vi "Pkg New.vi"(8 "error in (no error)":errorcluster, 10 "Package Name":string, 11 "Root Directory":path) -> (0 "error out":errorcluster, 3 "Created":path[](array[path]))   [LabVIEW 2018, in "Pkg.lvlib"]
uses:
  Pkg.lvlib
  <vilib>/ErrorRing/Error Ring.xnode
  <vilib>/Utility/error.llb/Error Cluster From Error Code.vi
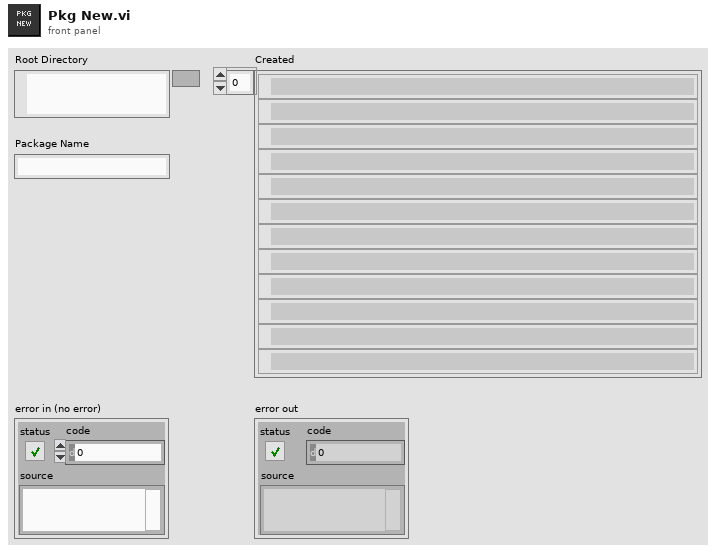
[diagram p1: front panel]
types:
  T1 = cluster{"RootDir":path, "PkgName":string, "PkgDir":path, "PkgBuildsDir":path, "PkgConfigsDir":path, "PkgDocsDir":path, "PkgLibDir":path, "PkgTestsDir":path, "PkgPackageIni":path, "PkgLibLvproj":path, "PkgLibSettingsIni":path, "PkgLibLvlib":path, "PkgLibVI":path}
  T2 = enum32{"invalid app kind", "Development System", "Run Time System", "Student Edition", "Embedded LabVIEW", "Evaluation", "Custom"}
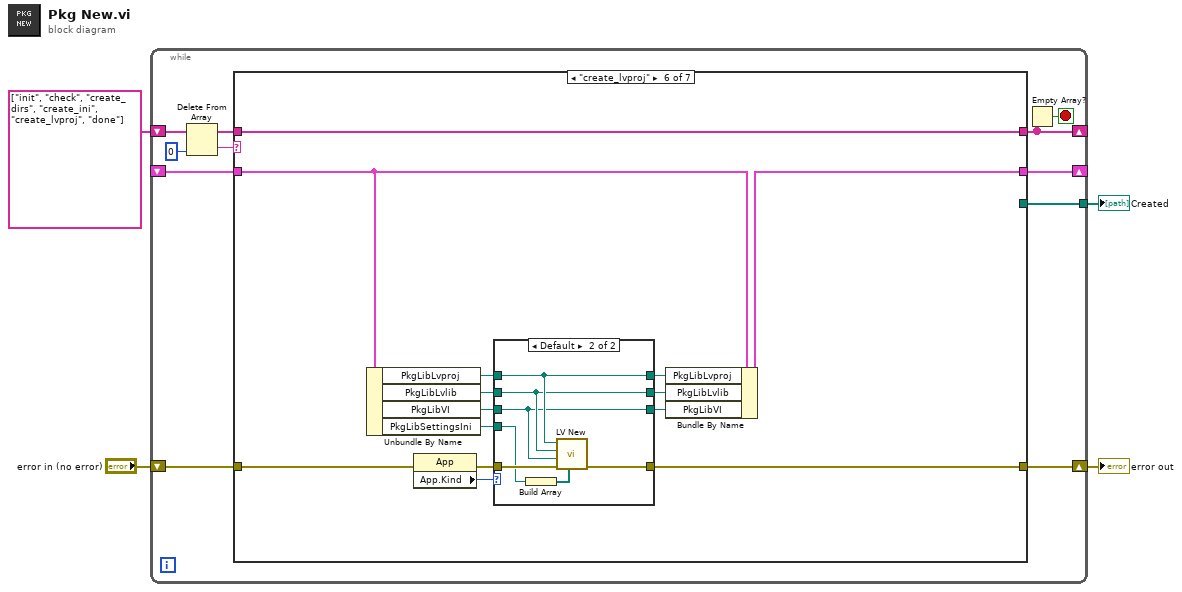
[diagram p0: block diagram]
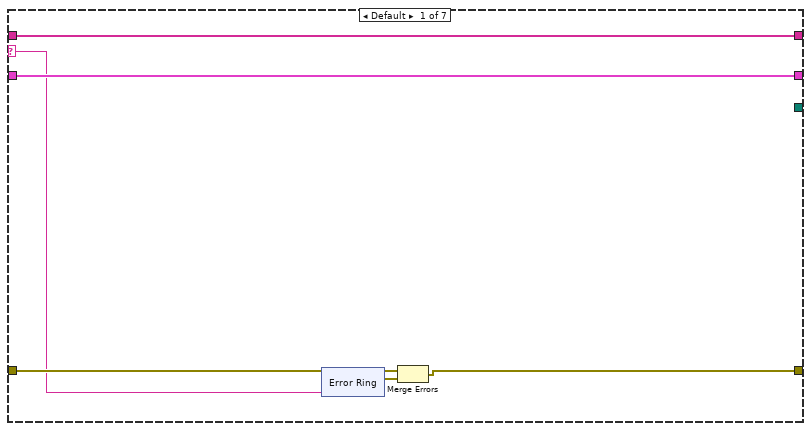
[diagram p2: hidden frame]
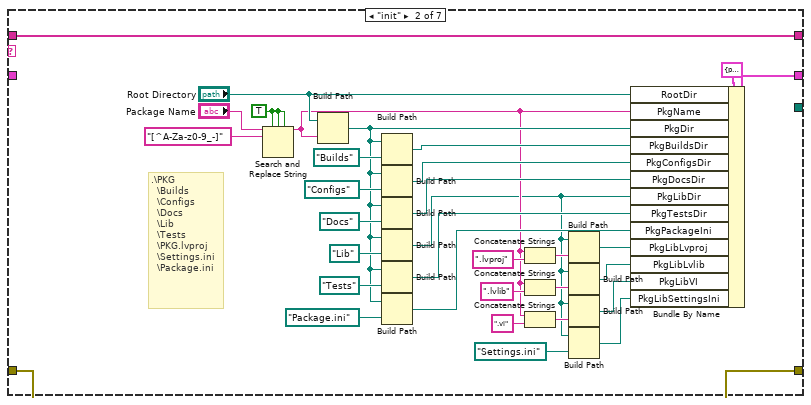
[diagram p3: hidden frame]
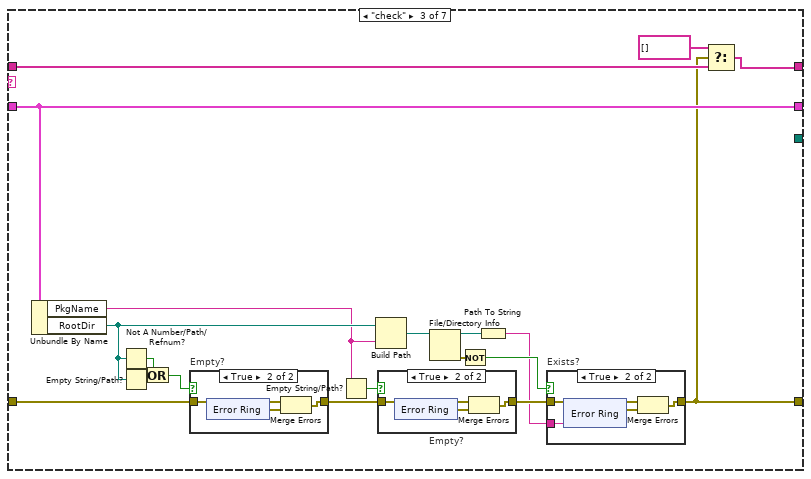
[diagram p4: hidden frame]
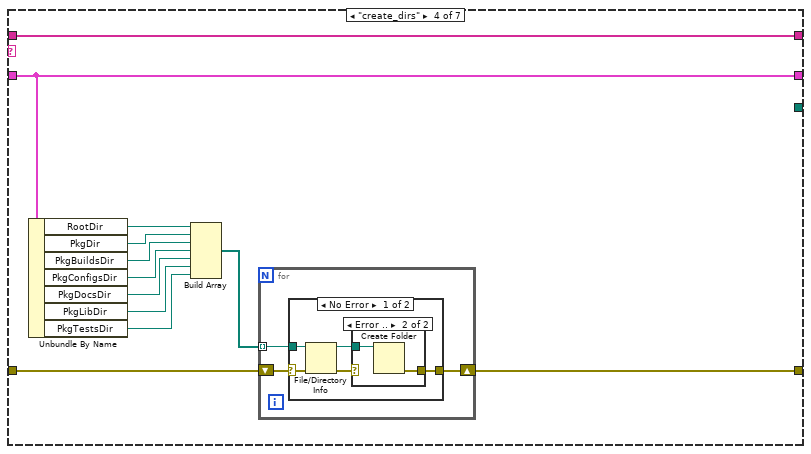
[diagram p8: hidden frame]
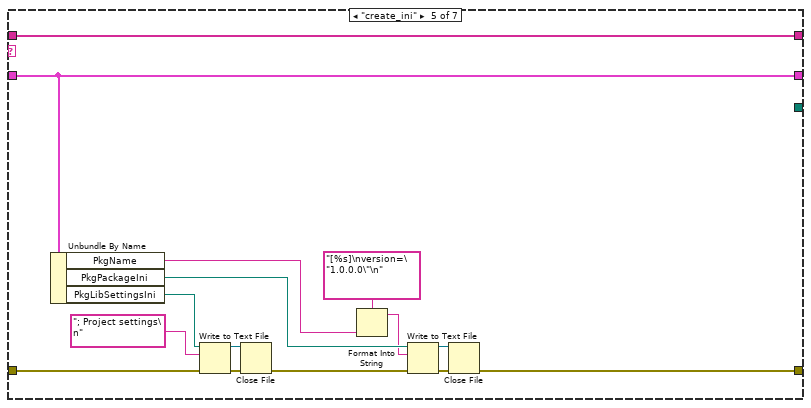
[diagram p11: hidden frame]
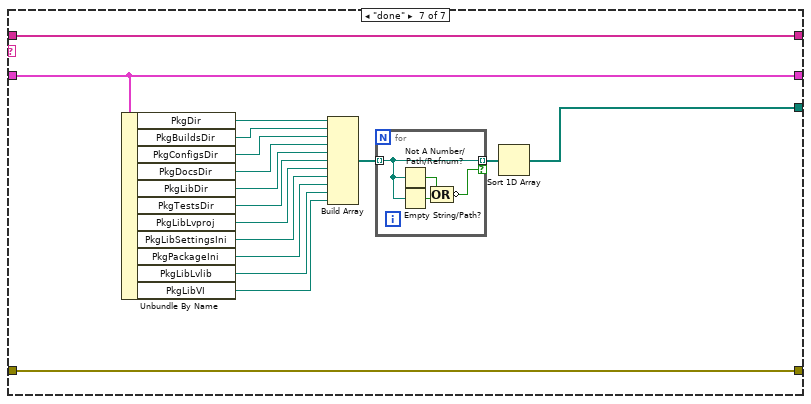
[diagram p13: hidden frame]
diagram:
  n1 = while {
    shift-right: [w7] -> _
    shift-left: string[] ["init", "check", "create_dirs", "create_ini", "create_lvproj", "done"] -> [w15]
    shift-right: [w9] -> _
    shift-left: _ -> [w8]
    shift-right: [w11] -> w3
    shift-left: "error in (no error)" -> [w10]
    tunnel: [w5] -> w1
    stop <- w6 stop-if-true
    n2 = Delete From Array(array=w15, index=0) -> (deleted portion=w12:string, array with subset deleted=w13:string[])  [unwired: 1 in]
    n3 = case shown="\"create_lvproj\"" w12 {
      selector: w12 -> [w16 _ _ _ _ _ _]
      tunnel: [w21 w61 w75 w122 w149 w163 w188] -> w7
      tunnel: w13 -> [w21 w61 w74 w122 w149 w163 w188]
      tunnel: [w18 w39 w64 w120 w139 w160 w187] -> w11
      tunnel: w10 -> [w19 w39 w80 w118 w148 w161 w187]
      tunnel: [w20 w59 w79 w121 w147 w154 w186] -> w9
      tunnel: w8 -> [w20 _ w79 w121 w147 w162 w186]
      tunnel: [_ _ _ _ _ _ w172] -> w5
      frame Default {
        n4 = xnode "Error Ring"("parameter 0"=w16) -> ("error out"=w17:errorcluster)
        n5 = Merge Errors(w19, w17) -> (w18:errorcluster)
      }
      frame "init" {
        w58 = TRUE ("replace all? (F)")
        # ".\\PKG\n  \\Builds\n  \\Configs\n  \\Docs\n  \\Lib\n  \\Tests\n  \\PKG.lvproj\n  \\Settings.ini\n  \\Package.ini"
        n6 = Search and Replace String(replace all?=w58, case sensitive?=w58, multiline?=w58, input string="Package Name", search string="[^A-Za-z0-9_-]") -> (result string=w32:string)  [unwired: 3 in, 3 out]
        n7 = Build Path(base path="Root Directory", name or relative path=w32) -> (appended path=w36:path)
        n8 = Build Path(base path=w36, name or relative path=path "Builds") -> (appended path=w49:path)
        n9 = Build Path(base path=w36, name or relative path=path "Configs") -> (appended path=w48:path)
        n10 = Build Path(base path=w36, name or relative path=path "Docs") -> (appended path=w47:path)
        n11 = Build Path(base path=w36, name or relative path=path "Lib") -> (appended path=w30:path)
        n12 = Build Path(base path=w36, name or relative path=path "Tests") -> (appended path=w46:path)
        n13 = Build Path(base path=w36, name or relative path=path "Package.ini") -> (appended path=w35:path)
        n14 = Concatenate Strings(w32, ".lvproj" ("string")) -> (w41:string)
        n15 = Concatenate Strings(w32, ".lvlib" ("string")) -> (w45:string)
        n16 = Concatenate Strings(w32, ".vi" ("string")) -> (w42:string)
        n17 = Build Path(base path=w30, name or relative path=w41) -> (appended path=w31:path)
        n18 = Build Path(base path=w30, name or relative path=w45) -> (appended path=w34:path)
        n19 = Build Path(base path=w30, name or relative path=w42) -> (appended path=w33:path)
        n20 = Build Path(base path=w30, name or relative path=path "Settings.ini") -> (appended path=w29:path)
        n21 = Bundle By Name(cluster=T1 {"RootDir"=path "", "PkgName"="", "PkgDir"=path "", "PkgBuildsDir"=path "", "PkgConfigsDir"=path "", "PkgDocsDir"=path "", "PkgLibDir"=path "", "PkgTestsDir"=path "", "PkgPackageIni"=path "", "PkgLibLvproj"=path "", "PkgLibSettingsIni"=path "", "PkgLibLvlib"=path "", "PkgLibVI"=path ""} ("StateData"), "RootDir"="Root Directory", "PkgName"=w32, "PkgDir"=w36, "PkgBuildsDir"=w49, "PkgConfigsDir"=w48, "PkgDocsDir"=w47, "PkgLibDir"=w30, "PkgTestsDir"=w46, "PkgPackageIni"=w35, "PkgLibLvproj"=w31, "PkgLibLvlib"=w34, "PkgLibVI"=w33, "PkgLibSettingsIni"=w29) -> (w59:T1)
      }
      frame "check" {
        n22 = Unbundle By Name(w79) -> ("PkgName"=w69:string, "RootDir"=w70:path)
        n23 = Not A Number/Path/Refnum?(number/path/refnum=w70) -> (NaN/Path/Refnum?=w77:bool)
        n24 = Empty String/Path?(string/path=w70) -> (empty?=w78:bool)
        n25 = Or(x=w77, y=w78) -> (x .or. y?=w73:bool)
        n26 = case "Empty?" shown="True" w73 {
          tunnel: w80 -> [w102 w105]
          tunnel: [w102 w103] -> w72
          frame False {
          }
          frame True {
            n27 = xnode "Error Ring"() -> ("error out"=w104:errorcluster)
            n28 = Merge Errors(w105, w104) -> (w103:errorcluster)
          }
        }
        n29 = Empty String/Path?(string/path=w69) -> (empty?=w71:bool)
        n30 = Build Path(base path=w70, name or relative path=w69) -> (appended path=w68:path)
        n31 = case "Empty?" shown="True" w71 {
          tunnel: w72 -> [w93 w96]
          tunnel: [w93 w94] -> w65
          frame False {
          }
          frame True {
            n32 = xnode "Error Ring"() -> ("error out"=w95:errorcluster)
            n33 = Merge Errors(w96, w95) -> (w94:errorcluster)
          }
        }
        n34 = File/Directory Info(path=w68) -> (path out=w63:path, error out=w67:errorcluster)  [unwired: 1 in, 5 out]
        n35 = Not(x=w67) -> (.not. x?=w66:bool)
        n36 = Path To String(path=w63) -> (string=w62:string)
        n37 = case "Exists?" shown="True" w66 {
          tunnel: w65 -> [w81 w85]
          tunnel: [w81 w83] -> w64
          tunnel: w62 -> [_ w82]
          frame False {
          }
          frame True {
            n38 = xnode "Error Ring"("parameter 0"=w82) -> ("error out"=w84:errorcluster)
            n39 = Merge Errors(w85, w84) -> (w83:errorcluster)
          }
        }
        n40 = Select(t=string[] [], s=w64, f=w74) -> (s? t:f=w75:string[])
      }
      frame "create_dirs" {
        n41 = Unbundle By Name(w121) -> ("RootDir"=w119:path, "PkgDir"=w116:path, "PkgBuildsDir"=w115:path, "PkgConfigsDir"=w114:path, "PkgDocsDir"=w113:path, "PkgLibDir"=w112:path, "PkgTestsDir"=w111:path)
        n42 = Build Array(w119, w116, w115, w114, w113, w112, w111) -> (w117:path[])
        n43 = for {
          tunnel: w117 -> [w124] mode=indexing
          shift-right: [w125] -> w120
          shift-left: w118 -> [w123]
          n44 = case shown="No Error" w123 {
            selector: w123 -> [w126 w134]
            tunnel: [w130 w134] -> w125
            tunnel: w124 -> [w129 _]
            frame No Error {
              n45 = File/Directory Info(path=w129, error in=w126) -> (path out=w128:path, error out=w127:errorcluster)  [unwired: 5 out]
              n46 = case shown="Error .." w127 {
                selector: w127 -> [w131 _]
                tunnel: [w131 w133] -> w130
                tunnel: w128 -> [_ w132]
                frame No Error {
                }
                frame Error {
                  n47 = Create Folder(path (use dialog)=w132) -> (error out=w133:errorcluster)  [unwired: 2 in, 2 out]
                }
              }
            }
            frame Error {
            }
          }
        }
      }
      frame "create_ini" {
        n48 = Unbundle By Name(w147) -> ("PkgName"=w136:string, "PkgPackageIni"=w138:path, "PkgLibSettingsIni"=w144:path)
        n49 = Write to Text File(file (use dialog)=w144, text="; Project settings\n", error in=w148) -> (refnum out=w145:refnum<file>, error out=w146:errorcluster)  [unwired: 1 in, 1 out]
        n50 = Close File(refnum=w145, error in=w146) -> (error out=w140:errorcluster)  [unwired: 1 out]
        n51 = Format Into String(format string="[%s]\nversion=\"1.0.0.0\"\n" ("text"), w136) -> (resulting string=w135:string)  [unwired: 2 in, 1 out]
        n52 = Write to Text File(file (use dialog)=w138, text=w135, error in=w140) -> (refnum out=w142:refnum<file>, error out=w141:errorcluster)  [unwired: 1 in, 1 out]
        n53 = Close File(refnum=w142, error in=w141) -> (error out=w139:errorcluster)  [unwired: 1 out]
      }
      frame "create_lvproj" {
        n54 = Unbundle By Name(w162) -> ("PkgLibLvproj"=w159:path, "PkgLibLvlib"=w158:path, "PkgLibVI"=w157:path, "PkgLibSettingsIni"=w150:path)
        n55 = property class="App"(error in=w161) -> (error out=w156:errorcluster, "App.Kind"=w155:T2)  [unwired: 1 in, 1 out]
        n56 = case shown="Default" w155 {
          tunnel: [w164 w171] -> w160
          tunnel: w159 -> [_ w169]
          tunnel: w158 -> [_ w168]
          tunnel: w157 -> [_ w167]
          tunnel: w156 -> [w164 w170]
          tunnel: [_ w169] -> w153
          tunnel: [_ w168] -> w152
          tunnel: [_ w167] -> w151
          tunnel: w150 -> [_ w166]
          frame "Run Time System" {
          }
          frame Default {
            n57 = Build Array(w166) -> (w165:path[])
            n58 = call "LV New.vi"("Misc Project Files"=w165, "error in (no error)"=w170, "VI"=w167, "Lvlib"=w168, "Lvproj"=w169) -> ("error out"=w171:errorcluster)  [unwired: 6 in]
          }
        }
        n59 = Bundle By Name(cluster=w162, "PkgLibLvproj"=w153, "PkgLibLvlib"=w152, "PkgLibVI"=w151) -> (w154:T1)
      }
      frame "done" {
        n60 = Unbundle By Name(w186) -> ("PkgDir"=w185:path, "PkgBuildsDir"=w184:path, "PkgConfigsDir"=w183:path, "PkgDocsDir"=w182:path, "PkgLibDir"=w181:path, "PkgTestsDir"=w180:path, "PkgLibLvproj"=w179:path, "PkgLibSettingsIni"=w178:path, "PkgPackageIni"=w177:path, "PkgLibLvlib"=w176:path, "PkgLibVI"=w175:path)
        n61 = Build Array(w185, w184, w183, w182, w181, w180, w179, w178, w177, w176, w175) -> (w174:path[])
        n62 = for {
          tunnel: w174 -> [w190] mode=indexing
          tunnel: [w190] -> w173 mode=indexing if=w189
          n63 = Not A Number/Path/Refnum?(number/path/refnum=w190) -> (NaN/Path/Refnum?=w191:bool)
          n64 = Empty String/Path?(string/path=w190) -> (empty?=w192:bool)
          n65 = Compound Arithmetic op=OR(w191, w192) -> (invert w189:bool)
        }
        n66 = Sort 1D Array(array=w173) -> (sorted array=w172:path[])
      }
    }
    n67 = Empty Array?(array=w7) -> (empty?=w6:bool)
  }
  "error out" <- w3
  "Created" <- w1
